vi "5492_IndexIndexes.vi"(8 "Shapes Found":dbl, 10 "Indexes":dbl[](array[numeric]), 11 "Full Data":dbl[](array[numeric])) -> (3 "Output Array":dbl[](array[numeric]))   [LabVIEW 2016]
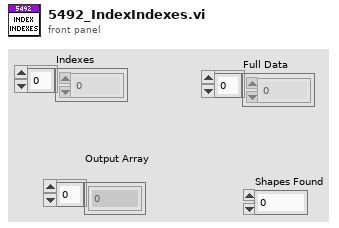
[diagram p1: front panel]
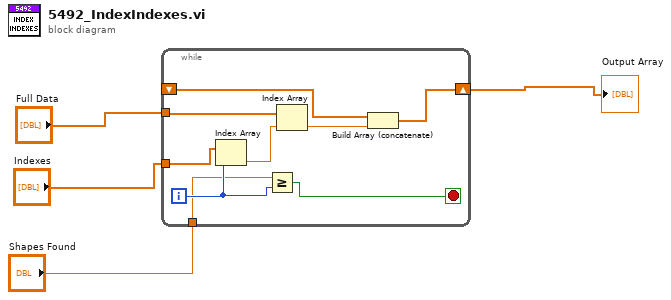
[diagram p0: block diagram]
diagram:
  n1 = while {
    tunnel: "Full Data" -> [w13]
    tunnel: "Indexes" -> [w11]
    shift-right: [w7] -> w1
    shift-left: _ -> [w6]
    tunnel: "Shapes Found" -> [w5]
    i -> [w10]
    stop <- w9 stop-if-true
    n2 = Index Array(array=w11, index=w10) -> (element=w12:dbl)
    n3 = Greater Or Equal?(x=w5, y=w10) -> (x >= y?=w9:bool)
    n4 = Index Array(array=w13, index=w12) -> (element=w8:dbl)
    n5 = Build Array (concatenate)(w6, w8) -> (w7:dbl[])
  }
  "Output Array" <- w1
